vi "TotalModifiedTx.vi"() -> ()   [LabVIEW 2012]
uses:
  <vilib>/addons/Modulation/Digital/General/MT Generate PSK System Parameters(M).vi
  <instrlib>/niUSRP/niUSRP Write Tx Data (CDB Cluster).vi
  <vilib>/addons/Modulation/niDMT.lvlib
panel:
  out "Numeric":u32
  out "output cluster":T1
  in  "Referance Cluster":T1={"Tx IQ Sampling\nRate [s/sec]"=500000.0, "Tx Frequency [Hz]"=2500000000.0, "Tx Gain [dB]"=0.0, "Tx Antenna"="TX1"} {"Tx Gain [dB]" format="%#.6p"; "Tx Frequency [Hz]" format="%#.6p"; "Tx IQ Sampling\nRate [s/sec]" format="%#.6p"}
  in  "Frequency of\noperation":dbl
  out "Required Power":dbl
  out "String":string
  out "millisecond timer value":u32
  out "Entering into 2nd \n          Loop":string
  out "Symbol Rate\n[symbols/sec]":dbl=25000.0 format="%#.6p"
  in  "BPSK System Parameters 9":T2={"Samples per Symbol"=8, "symbol map"=[], "Differential PSK"=enum."disable", "PSK type"=0} caption="BPSK System Parameters" {"PSK type" items=["normal", "shifted", "offset"]; "symbol map" format="%.3f"}
  in  "BPSK System Parameters 8":T2={"Samples per Symbol"=8, "symbol map"=[], "Differential PSK"=enum."disable", "PSK type"=0} caption="BPSK System Parameters" {"PSK type" items=["normal", "shifted", "offset"]; "symbol map" format="%.3f"}
  in  "BPSK System Parameters 7":T2={"Samples per Symbol"=8, "symbol map"=[], "Differential PSK"=enum."disable", "PSK type"=0} caption="BPSK System Parameters" {"PSK type" items=["normal", "shifted", "offset"]; "symbol map" format="%.3f"}
  in  "BPSK System Parameters 6":T2={"Samples per Symbol"=8, "symbol map"=[], "Differential PSK"=enum."disable", "PSK type"=0} caption="BPSK System Parameters" {"PSK type" items=["normal", "shifted", "offset"]; "symbol map" format="%.3f"}
  in  "BPSK System Parameters 5":T2={"Samples per Symbol"=8, "symbol map"=[], "Differential PSK"=enum."disable", "PSK type"=0} caption="BPSK System Parameters" {"PSK type" items=["normal", "shifted", "offset"]; "symbol map" format="%.3f"}
  in  "BPSK System Parameters 4":T2={"Samples per Symbol"=8, "symbol map"=[], "Differential PSK"=enum."disable", "PSK type"=0} caption="BPSK System Parameters" {"PSK type" items=["normal", "shifted", "offset"]; "symbol map" format="%.3f"}
  in  "BPSK System Parameters 3":T2={"Samples per Symbol"=8, "symbol map"=[], "Differential PSK"=enum."disable", "PSK type"=0} caption="BPSK System Parameters" {"PSK type" items=["normal", "shifted", "offset"]; "symbol map" format="%.3f"}
  in  "Tab Control":T3(tab)
  in  "Enter control signal (1,2 or 3)":string
  in  "Packet Parameters":T4={"Guard Bits "=30, "Sync Bits"=20, "Message Bits"=128}
  in  "Packet Pad \n[samples]":i32=200
  in  "Blank Frame \n[samples]":i32=500
  out "Number of Packets in Message":i32=46
  in  "PN sequence order\nfor Sync Bits":i32=31 caption="PN sequence order (9)"
  in  "Packet Repeat":i32=2
  in  "Pulse Shaping Filter Parameters":T5={"Alpha"=0.5, "Filter Length"=6, "TX Filter"=enum."Root Raised Cos"} caption="Pulse Shaping Filter" {"Alpha" format="%.2f"}
  out "Actual Tx Parameters":T1={"Tx IQ Sampling\nRate [s/sec]"=200000.0, "Tx Frequency [Hz]"=2500000000.0, "Tx Gain [dB]"=0.0, "Tx Antenna"="TX1"} {"Tx Gain [dB]" format="%#.6p"; "Tx Frequency [Hz]" format="%#.6p"; "Tx IQ Sampling\nRate [s/sec]" format="%#.6p"}
  in  "USRP IP address":refnum<k15>="192.168.10.2"
  out "error out":errorcluster
  in  "Queue Length":i32=10
  out "Transmission\n       Stop":bool
  in  "end of data?":bool
  out "Constellation Graph":T6(graph)
  in  "autoscale":bool
  out "millisecond timer value 2":u32
  out "x = y?":bool
  out "Transmission\n      Time":bool
  out "error out 2":errorcluster
  out "Message Text 3":string="Two roads diverged in a yellow wood,\nAnd sorry I could not travel both\nAnd be one traveler, long I stood\nAnd looked down one as far as I could\nTo where it bent in the undergrowth.\n\nThen took the other, as just as fair,\nAnd having perhaps the better claim,\nBecause it was grassy and wanted wear;\nThough as for that the passing there\nHad worn them really about the same.\n\nAnd both that morning equally lay\nIn leaves no step had trodden black.\nOh, I kept the first for another day!\nYet knowing how way leads on to way,\nI doubted if I should ever come back.\n\nI shall be telling this with a sigh\nSomewhere ages and ages hence:\nTwo roads diverged in a wood, and I--\nI took the one less traveled by,\nAnd that has made all the difference.\n"
  out "M-PSK (4)":i32
  # "Guard\nBand"
  # "Sync\nSeq"
  # "Packet\nNumber"
  # "Pad\nData"
  # "Blank\nFrame"
  # "Data"
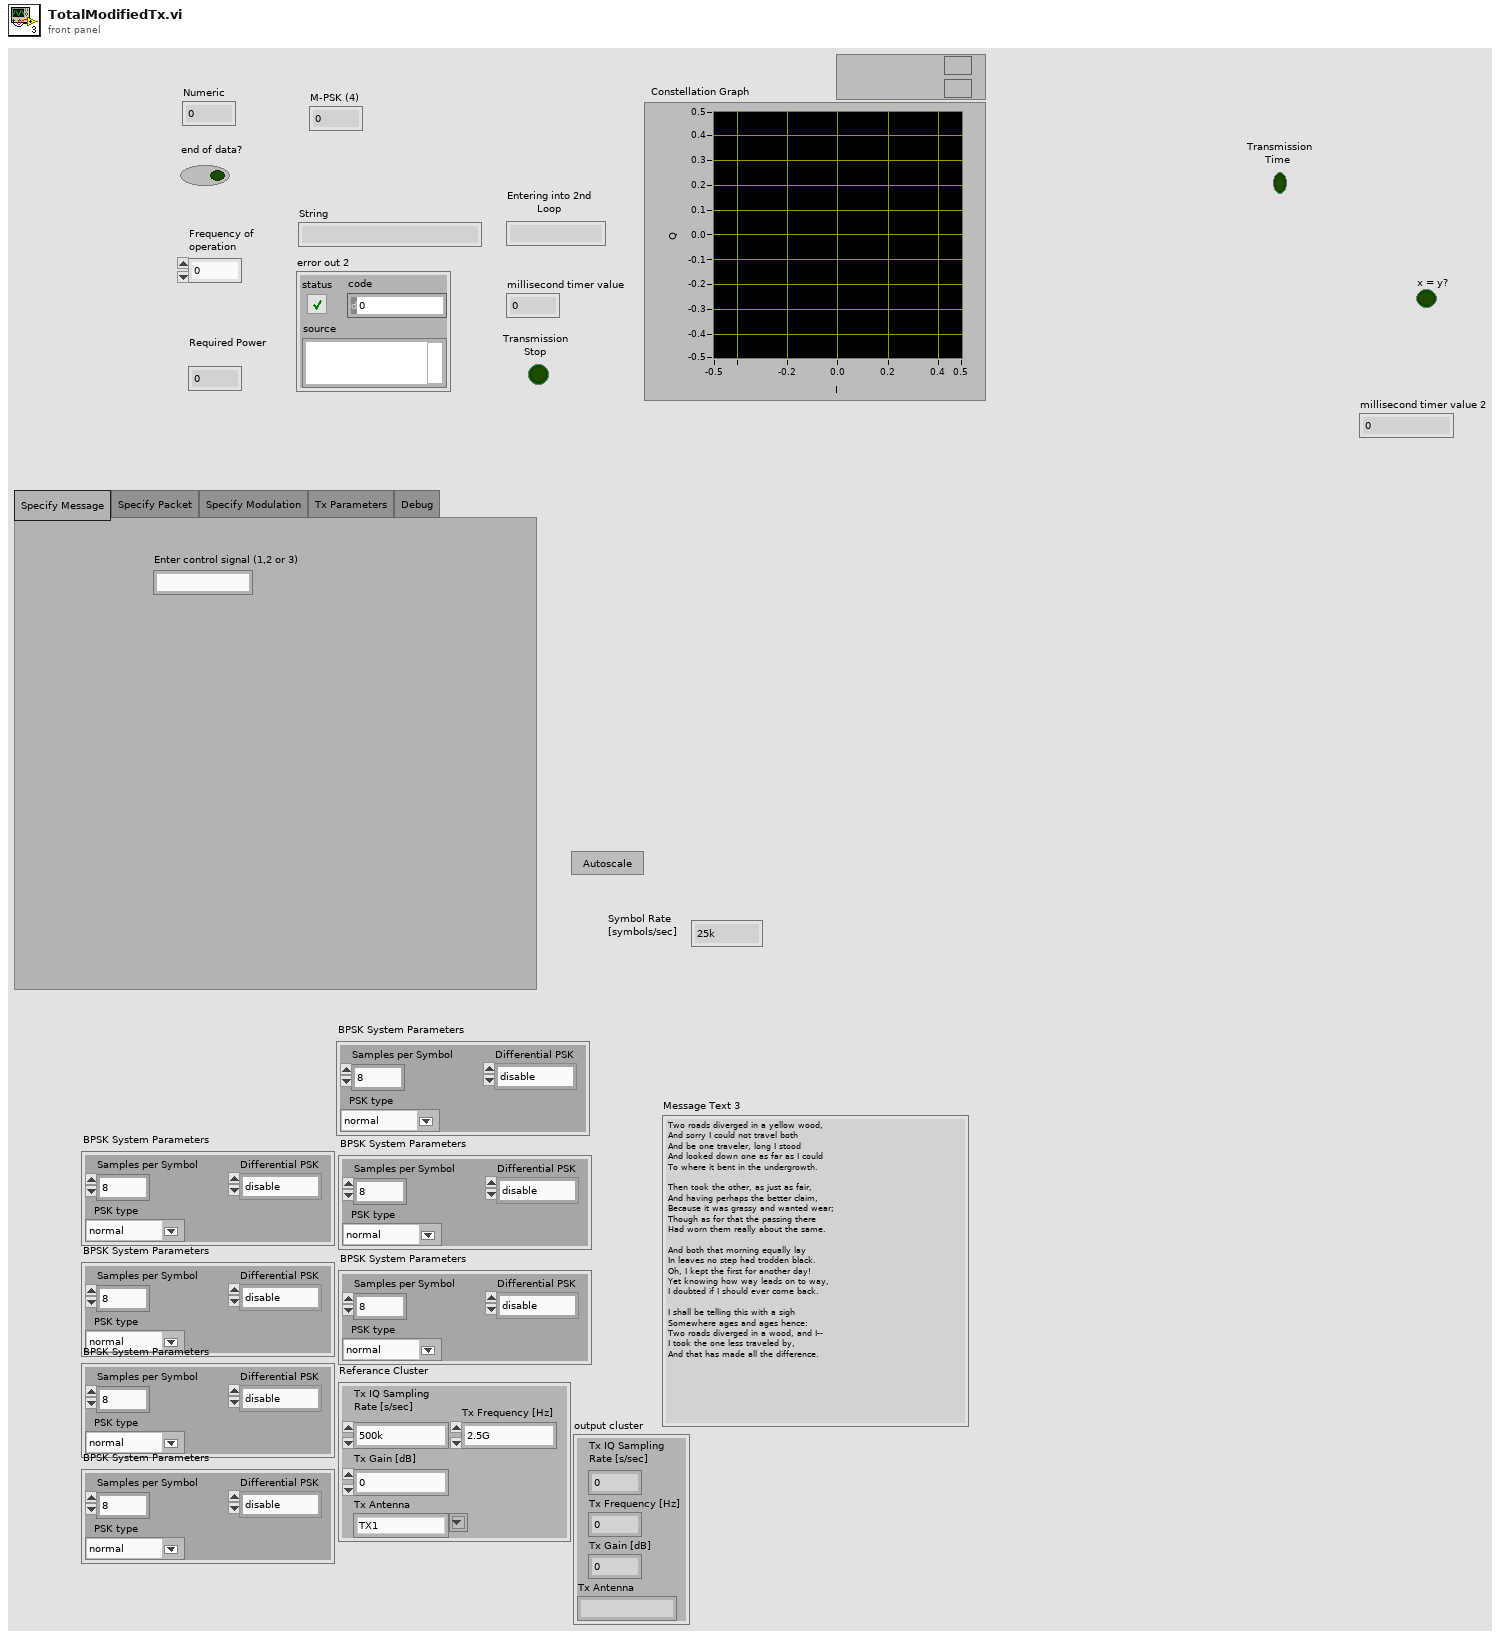
[diagram p1: front panel]
types:
  T1 = cluster{"Tx IQ Sampling\nRate [s/sec]":dbl, "Tx Frequency [Hz]":dbl, "Tx Gain [dB]":dbl, "Tx Antenna":string}
  T2 = cluster{"Samples per Symbol":i32, "symbol map":cdb[], "Differential PSK":enum16{"disable", "enable"}, "PSK type":u16}
  T3 = enum32{"Specify Message", "Specify Packet", "Specify Modulation", "Tx Parameters", "Debug"}
  T4 = cluster{"Guard Bits ":i32, "Sync Bits":i32, "Message Bits":i32}
  T5 = cluster{"Alpha":dbl, "Filter Length":i32, "TX Filter":enum16{"none", "Raised Cosine", "Root Raised Cos", "Gaussian"}}
  T6 = cluster{"Decimated Array":dbl[], "Decimated Array":dbl[]}[]
  T7 = cluster{"samples per symbol (16)":i32, "symbol map":cdb[], "differential PSK":enum16{"disable", "enable"}, "PSK type":u16}
  T8 = cluster{"s? t:f":cluster{"t0":dbl, "dt":dbl, "Y":cdb[]}, i32}
  T9 = cluster{"output complex waveform":cluster{"t0":dbl, "dt":dbl, "Y":cdb[]}, i32}
  T10 = cluster{"constellation":dbl[], "oversampled data":dbl[]}[]
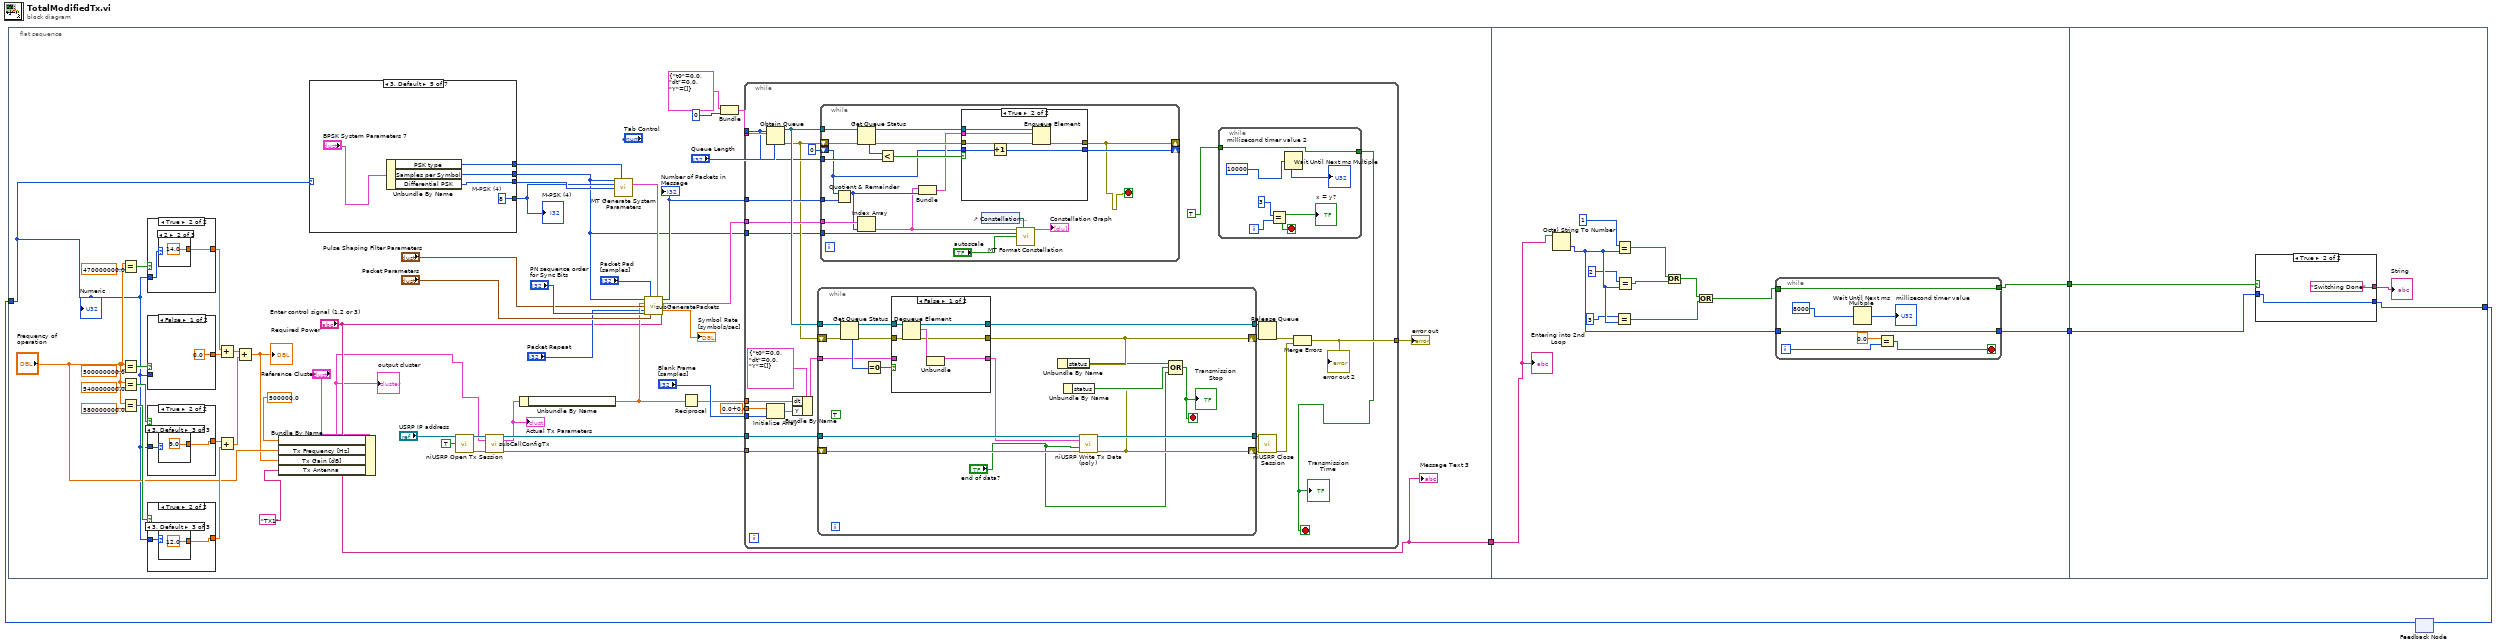
[diagram p0: block diagram]
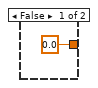
[diagram p2: hidden frame]
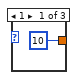
[diagram p3: hidden frame]
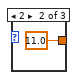
[diagram p4: hidden frame]
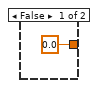
[diagram p5: hidden frame]
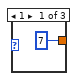
[diagram p6: hidden frame]
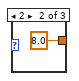
[diagram p7: hidden frame]
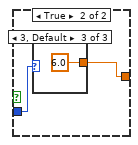
[diagram p8: hidden frame]
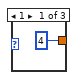
[diagram p9: hidden frame]
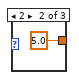
[diagram p10: hidden frame]
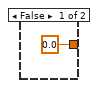
[diagram p11: hidden frame]
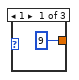
[diagram p12: hidden frame]
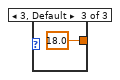
[diagram p13: hidden frame]
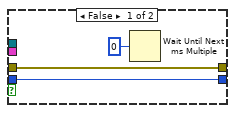
[diagram p14: hidden frame]
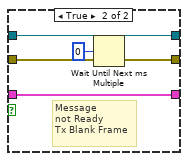
[diagram p15: hidden frame]
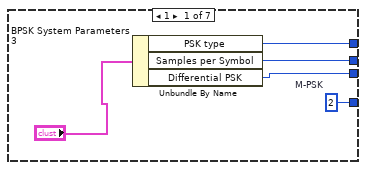
[diagram p16: hidden frame]
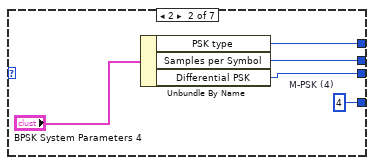
[diagram p17: hidden frame]
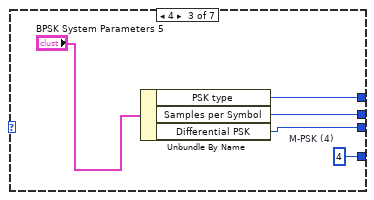
[diagram p18: hidden frame]
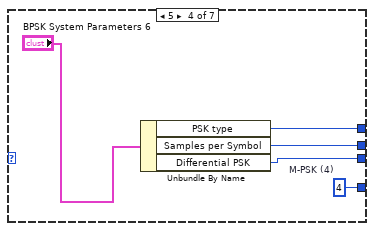
[diagram p19: hidden frame]
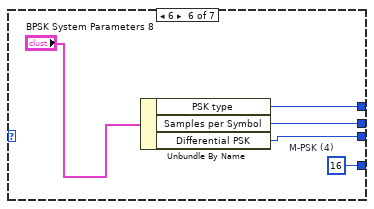
[diagram p20: hidden frame]
diagram:
  n1 = flat-sequence {
    tunnel: ["Enter control signal (1,2 or 3)"] -> w5
    tunnel: w1 -> [w6]
    tunnel: w5 -> [w203]
    tunnel: [w205] -> w4
    tunnel: [w204] -> w3
    tunnel: w4 -> [w224]
    tunnel: w3 -> [w223]
    tunnel: [w222] -> w2
    frame #0 {
      n2 = Equal?(x="Frequency of\noperation", y=470000000.0) -> (x = y?=w13:bool)
      n3 = Equal?(x="Frequency of\noperation", y=500000000.0) -> (x = y?=w14:bool)
      n4 = Equal?(x="Frequency of\noperation", y=540000000.0) -> (x = y?=w15:bool)
      n5 = Equal?(x="Frequency of\noperation", y=580000000.0) -> (x = y?=w16:bool)
      n6 = case shown="True" w13 {
        tunnel: [0.0 w76] -> w24
        tunnel: w6 -> [_ w77]
        frame False {
        }
        frame True {
          n7 = case shown="2" w77 {
            tunnel: [9 14.0 18.0] -> w76
            frame 1 {
            }
            frame 2 {
            }
            frame 3, Default {
            }
          }
        }
      }
      n8 = case shown="False" w14 {
        tunnel: [0.0 w70] -> w23
        tunnel: w6 -> [_ w71]
        frame False {
        }
        frame True {
          n9 = case shown="3, Default" w71 {
            tunnel: [4 5.0 6.0] -> w70
            frame 1 {
            }
            frame 2 {
            }
            frame 3, Default {
            }
          }
        }
      }
      n10 = case shown="True" w15 {
        tunnel: [0.0 w64] -> w22
        tunnel: w6 -> [_ w65]
        frame False {
        }
        frame True {
          n11 = case shown="3, Default" w65 {
            tunnel: [7 8.0 9.0] -> w64
            frame 1 {
            }
            frame 2 {
            }
            frame 3, Default {
            }
          }
        }
      }
      n12 = case shown="True" w16 {
        tunnel: [0.0 w58] -> w21
        tunnel: w6 -> [_ w59]
        frame False {
        }
        frame True {
          n13 = case shown="3, Default" w59 {
            tunnel: [10 11.0 12.0] -> w58
            frame 1 {
            }
            frame 2 {
            }
            frame 3, Default {
            }
          }
        }
      }
      n14 = Add(x=w24, y=w23) -> (x+y=w26:dbl)
      n15 = Add(x=w22, y=w21) -> (x+y=w25:dbl)
      n16 = Add(x=w26, y=w25) -> (x+y=w10:dbl)
      "Required Power" <- w10
      n17 = Bundle By Name(cluster="Referance Cluster", "Tx IQ Sampling\nRate [s/sec]"=500000.0, "Tx Frequency [Hz]"="Frequency of\noperation", "Tx Gain [dB]"=w10, "Tx Antenna"="TX1") -> (w8:T1)
      "output cluster" <- w8
      n18 = case shown="3, Default" w6 {
        tunnel: [w169 w174 w181 w186 w191 w197 w200] -> w30
        tunnel: [w170 w175 w180 w185 w190 w196 w201] -> w56
        tunnel: [w172 w177 w182 w187 w189 w195 0 ("M-PSK (4)")] -> w47
        tunnel: [w171 w176 w179 w184 w192 w194 w202] -> w36
        frame 1 {
          w172 = 2  # M-PSK
          n19 = Unbundle By Name("BPSK System Parameters 3") -> ("PSK type"=w171:u16, "Samples per Symbol"=w169:i32, "Differential PSK"=w170:enum16{"disable", "enable"})
        }
        frame 2 {
          w177 = 4  # M-PSK (4)
          n20 = Unbundle By Name("BPSK System Parameters 4") -> ("PSK type"=w176:u16, "Samples per Symbol"=w174:i32, "Differential PSK"=w175:enum16{"disable", "enable"})
        }
        frame 4 {
          w182 = 4  # M-PSK (4)
          n21 = Unbundle By Name("BPSK System Parameters 5") -> ("PSK type"=w179:u16, "Samples per Symbol"=w181:i32, "Differential PSK"=w180:enum16{"disable", "enable"})
        }
        frame 5 {
          w187 = 4  # M-PSK (4)
          n22 = Unbundle By Name("BPSK System Parameters 6") -> ("PSK type"=w184:u16, "Samples per Symbol"=w186:i32, "Differential PSK"=w185:enum16{"disable", "enable"})
        }
        frame 3, Default {
          w189 = 8  # M-PSK (4)
          n23 = Unbundle By Name("BPSK System Parameters 7") -> ("PSK type"=w192:u16, "Samples per Symbol"=w191:i32, "Differential PSK"=w190:enum16{"disable", "enable"})
        }
        frame 6 {
          w195 = 16  # M-PSK (4)
          n24 = Unbundle By Name("BPSK System Parameters 8") -> ("PSK type"=w194:u16, "Samples per Symbol"=w197:i32, "Differential PSK"=w196:enum16{"disable", "enable"})
        }
        frame 7 {
          n25 = Unbundle By Name("BPSK System Parameters 9") -> ("PSK type"=w202:u16, "Samples per Symbol"=w200:i32, "Differential PSK"=w201:enum16{"disable", "enable"})
        }
      }
      "M-PSK (4)" <- w47
      n26 = call <instrlib>:"niUSRP Open Tx Session.vi"("device names"="USRP IP address", "reset"=TRUE) -> ("session handle out"=w40:refnum<k15>, "error out"=w39:errorcluster)  [unwired: 12 in]
      n27 = call "subCallConfigTx.vi"("session handle"=w40, "Tx Parameters"=w8, "error in"=w39) -> ("session handle out"=w46:refnum<k15>, "Actual Tx Parameters"=w45:T1, "error out"=w49:errorcluster)  [unwired: 10 in]
      "Actual Tx Parameters" <- w45
      n28 = Unbundle By Name(w45) -> ("Tx IQ Sampling\nRate [s/sec]"=w31:dbl)
      n29 = call-poly <vilib>:"MT Generate System Parameters.vi"("samples per symbol (16)"=w30, "PSK type"=w36, "M-PSK (4)"=w47, "differential PSK"=w56) -> ("PSK system parameters"=w37:T7)  [unwired: 9 in, 2 out]
      n30 = call "subGeneratePackets.vi"("Samples per Symbol"=w30, "Packet Pad \n[samples]"="Packet Pad \n[samples]", "PSK system parameters"=w37, "Tx IQ Sampling\nRate [s/sec]"=w31, "Pulse Shaping Filter Parameters"="Pulse Shaping Filter Parameters", "Packet Repeat"="Packet Repeat", "PN sequence order\nfor Sync Bits"="PN sequence order\nfor Sync Bits", "Packet Parameters"="Packet Parameters", "Message Text"="Enter control signal (1,2 or 3)") -> ("Number of Packets"=w44:i32, "Packets"=w50:cluster{"t0":dbl, "dt":dbl, "Y":cdb[]}[], "Symbol Rate"=→"Symbol Rate\n[symbols/sec]":dbl)  [unwired: 4 in]
      "Number of Packets in Message" <- w44
      n31 = Reciprocal(x=w31) -> (1/x=w48:dbl)
      n32 = Bundle("s? t:f"=cluster{"t0":dbl, "dt":dbl, "Y":cdb[]} {"t0"=0.0, "dt"=0.0, "Y"=[]}, 0) -> (w52:T8)  [unwired: 1 in]
      n33 = while {
        tunnel: cdb 0.0+0.0i ("element") -> [w105]
        tunnel: "Blank Frame \n[samples]" -> [w104]
        tunnel: w52 -> [w98]
        tunnel: "Queue Length" -> [w96]
        tunnel: w50 -> [w95]
        tunnel: w49 -> [w94]
        tunnel: w48 -> [w91]
        tunnel: w46 -> [w90]
        tunnel: w44 -> [w89]
        tunnel: [w84] -> w35
        tunnel: w30 -> [w83]
        stop <- w81 stop-if-true
        n34 = Obtain Queue(max queue size (-1, unlimited)=w96, element data type=w98) -> (queue out=w103:refnum<queue>, error out=w87:errorcluster)  [unwired: 3 in, 1 out]
        n35 = Initialize Array(w105, w104) -> (w102:cdb[])
        n36 = Bundle By Name(cluster=cluster{"t0":dbl, "dt":dbl, "Y":cdb[]} {"t0"=0.0, "dt"=0.0, "Y"=[]} ("s? t:f"), "dt"=w91, "Y"=w102) -> (w101:cluster{"t0":dbl, "dt":dbl, "Y":cdb[]})
        n37 = while {
          tunnel: w90 -> [w148]
          shift-right: [w145] -> w93
          shift-left: w94 -> [w149]
          tunnel: w103 -> [w157]
          tunnel: w101 -> [w154]
          tunnel: [w153] -> w100
          tunnel: [w147] -> w92
          shift-right: [w144] -> w99
          shift-left: w87 -> [w150]
          stop <- w141 stop-if-true
          (unwired) TRUE
          n38 = Get Queue Status(queue=w157, error in (no error)=w150) -> (queue out=w152:refnum<queue>, error out=w151:errorcluster, # elements in queue=w156:i32)  [unwired: 1 in, 5 out]
          n39 = Equal To 0?(x=w156) -> (x = 0?=w155:bool)
          n40 = case shown="False" w155 {
            tunnel: w154 -> [_ w167]
            tunnel: [w159 w167] -> w142
            tunnel: [w163 w165] -> w153
            tunnel: [w158 w166] -> w144
            tunnel: w152 -> [w162 w165]
            tunnel: w151 -> [w161 w166]
            frame False {
              n41 = Dequeue Element(queue=w162, error in (no error)=w161) -> (queue out=w163:refnum<queue>, element=w160:T8, error out=w158:errorcluster)  [unwired: 1 in, 1 out]
              n42 = Unbundle(w160) -> ("s? t:f"=w159:cluster{"t0":dbl, "dt":dbl, "Y":cdb[]})  [unwired: 1 out]
            }
            frame True {
              # "Message\nnot Ready\nTx Blank Frame"
              n43 = Wait Until Next ms Multiple(millisecond multiple=u32 0) -> ()  [unwired: 1 out]
            }
          }
          n44 = Unbundle By Name(w144) -> ("status"=w143:bool)
          n45 = call-poly <instrlib>:"niUSRP Write Tx Data (poly).vi"("session handle"=w148, "data"=w142, "end of data?"="end of data?", "error in (no error)"=w149) -> ("session handle out"=w147:refnum<k15>, "error out"=w145:errorcluster)  [unwired: 10 in]
          n46 = Unbundle By Name(w145) -> ("status"=w146:bool)
          n47 = Compound Arithmetic op=OR(w143, w146, "end of data?") -> (w141:bool)
          "Transmission\n       Stop" <- w141
        }
        n48 = while {
          tunnel: w103 -> [w130]
          shift-right: [w123] -> _
          shift-left: 0 -> [w119]
          tunnel: w95 -> [w120]
          tunnel: w96 -> [w122]
          tunnel: w89 -> [w121]
          shift-right: [w112] -> _
          shift-left: w87 -> [w125]
          tunnel: w83 -> [w115]
          stop <- w112 stop-if-true
          n49 = Quotient & Remainder(x=w119, y=w121) -> (x-y*floor(x/y)=w118:i32)  [unwired: 1 out]
          n50 = Index Array(array=w120, index=w118) -> (element=w113:cluster{"t0":dbl, "dt":dbl, "Y":cdb[]})
          n51 = Get Queue Status(queue=w130, error in (no error)=w125) -> (queue out=w129:refnum<queue>, error out=w126:errorcluster, # elements in queue=w128:i32)  [unwired: 1 in, 5 out]
          n52 = Less?(x=w128, y=w122) -> (x < y?=w127:bool)
          n53 = Bundle("output complex waveform"=w113, w118) -> (w124:T9)  [unwired: 1 in]
          n54 = case shown="True" w127 {
            tunnel: w126 -> [w131 w139]
            tunnel: w129 -> [_ w138]
            tunnel: [w131 w137] -> w112
            tunnel: w124 -> [_ w136]
            tunnel: w119 -> [w133 w135]
            tunnel: [w133 w134] -> w123
            frame False {
              n55 = Wait Until Next ms Multiple(millisecond multiple=u32 0) -> ()  [unwired: 1 out]
            }
            frame True {
              n56 = Increment(x=w135) -> (x+1=w134:i32)
              n57 = Enqueue Element(queue=w138, element=w136, error in (no error)=w139) -> (error out=w137:errorcluster)  [unwired: 1 in, 2 out]
            }
          }
          n58 = control-ref of="Constellation Graph"() -> (w116:refnum<vi>)
          n59 = call <vilib>:"MT Format Constellation.vi"("waveform"=w113, "constellation reference"=w116, "samples per symbol"=w115, "autoscale"="autoscale") -> ("constellation graph"=→"Constellation Graph":T10)  [unwired: 1 in, 10 out]
        }
        n60 = while {
          tunnel: TRUE -> [w111]
          tunnel: [w111] -> w81
          i -> [w109]
          stop <- w108 stop-if-true
          n61 = Equal?(x=3, y=w109) -> (x = y?=w108:bool)
          "x = y?" <- w108
          n62 = Wait Until Next ms Multiple(millisecond multiple=u32 10000) -> (millisecond timer value=→"millisecond timer value 2":u32)
        }
        "Transmission\n      Time" <- w81
        n63 = Release Queue(queue=w100, error in (no error)=w99) -> (error out=w86:errorcluster)  [unwired: 3 out]
        n64 = call <instrlib>:"niUSRP Close Session.vi"("session handle"=w92, "error in (no error)"=w93) -> ("error out"=w85:errorcluster)  [unwired: 13 in]
        n65 = Merge Errors(w86, w85) -> (w84:errorcluster)
        "error out 2" <- w84
      }
      "error out" <- w35
      "Message Text 3" <- "Enter control signal (1,2 or 3)"
      "Numeric" <- w6
    }
    frame #1 {
      n66 = Octal String To Number(4:w203) -> (0:w209:u32)  [unwired: 2 in, 1 out]
      n67 = Equal?(x=3, y=w209) -> (x = y?=w211:bool)
      n68 = Equal?(x=1, y=w209) -> (x = y?=w214:bool)
      n69 = Equal?(x=2, y=w209) -> (x = y?=w213:bool)
      n70 = Or(x=w214, y=w213) -> (x .or. y?=w212:bool)
      n71 = Or(x=w212, y=w211) -> (x .or. y?=w210:bool)
      n72 = while {
        tunnel: w210 -> [w220]
        tunnel: [w220] -> w205
        tunnel: w209 -> [w219]
        tunnel: [w219] -> w204
        i -> [w217]
        stop <- w216 stop-if-true
        n73 = Wait Until Next ms Multiple(millisecond multiple=u32 8000) -> (millisecond timer value=→"millisecond timer value":u32)
        n74 = Equal?(x=0.0, y=w217) -> (x = y?=w216:bool)
      }
      "Entering into 2nd \n          Loop" <- w203
    }
    frame #2 {
      n75 = case shown="True" w224 {
        tunnel: ["Not Done" "Switching Done"] -> w225
        tunnel: [_ w227] -> w222
        tunnel: w223 -> [_ w227]
        frame False {
        }
        frame True {
        }
      }
      "String" <- w225
    }
  }
  n76 = feedback #1() -> (w1:u32)  [unwired: 1 in]
  n77 = feedback-in #1(w2) -> ()
